vi "add setting.vi"(6 "replace if found?(T)":bool, 8 "error in (no error)":errorcluster, 9 "user settings":variant, 10 "id":string, 11 "DSFConfiguration in":refnum<class "DSFConfiguration.lvclass">) -> (0 "error out":errorcluster, 1 "found?":bool, 3 "DSFConfiguration out":refnum<class "DSFConfiguration.lvclass">)   [LabVIEW 2017, in "DSFConfiguration.lvclass"]
uses:
  DSFConfiguration.lvclass
  DSFConfiguration.lvclass/DSFConfiguration.ctl
  DSFPluginSettings/DSFPluginSettings.lvclass
  <vilib>/Utility/error.llb/Error Cluster From Error Code.vi
  <vilib>/ErrorRing/Error Ring.xnode
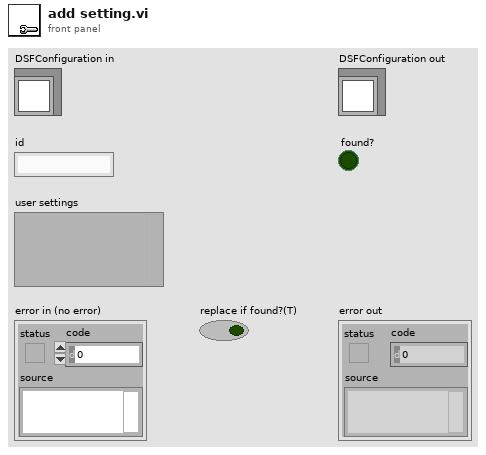
[diagram p1: front panel]
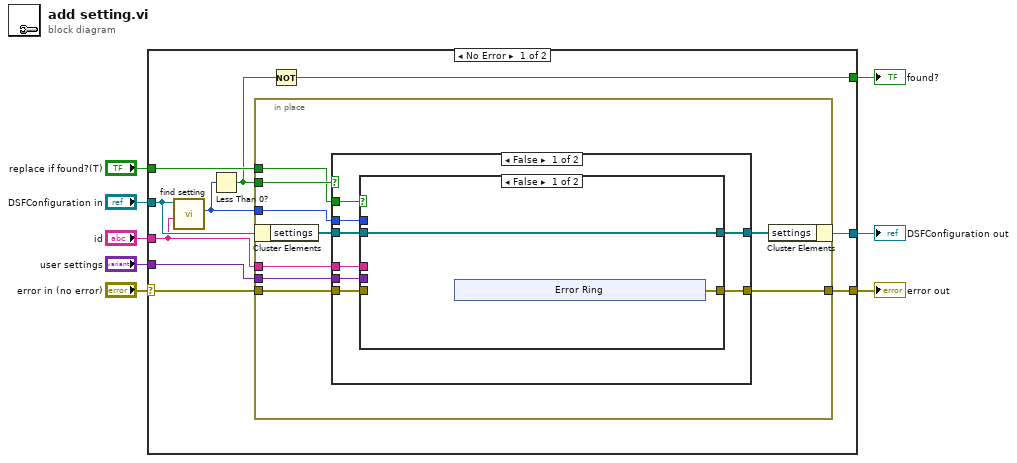
[diagram p0: block diagram]
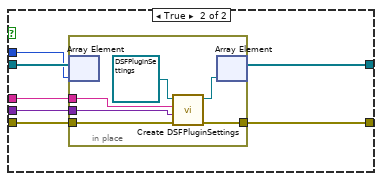
[diagram p2: hidden frame]
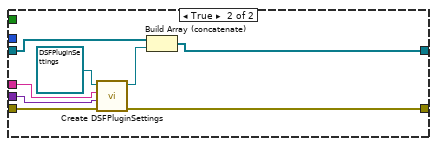
[diagram p3: hidden frame]
diagram:
  n1 = case shown="No Error" "error in (no error)" {
    selector: "error in (no error)" -> [w12 w64]
    tunnel: [w11 w64] -> w7
    tunnel: [w15 w63] -> w5
    tunnel: "DSFConfiguration in" -> [w18 w63]
    tunnel: "replace if found?(T)" -> [w17 _]
    tunnel: "id" -> [w14 _]
    tunnel: "user settings" -> [w13 _]
    tunnel: [w9 _] -> w1
    frame No Error {
      n2 = call "find setting.vi"("settings id"=w14, "DSFConfiguration in"=w18) -> ("index"=w16:i32)  [unwired: 9 in]
      n3 = Less Than 0?(x=w16) -> (x < 0?=w10:bool)
      n4 = in-place {
        in-place-border: w10 -> [w26]
        in-place-border: w14 -> [w25]
        in-place-border: w17 -> [w23]
        in-place-border: w16 -> [w22]
        in-place-border: w13 -> [w21]
        in-place-border: w12 -> [w20]
        in-place-border: [w19] -> w11
        n5 = in-place-cluster #1(w18) -> ("settings"=w27:refnum<class "DSFPluginSettings.lvclass">[])
        n6 = case shown="False" w26 {
          tunnel: w27 -> [w35 w62]
          tunnel: w25 -> [w32 w59]
          tunnel: [w31 w61] -> w24
          tunnel: w23 -> [w34 _]
          tunnel: w22 -> [w33 _]
          tunnel: w21 -> [w30 w58]
          tunnel: w20 -> [w29 w57]
          tunnel: [w28 w55] -> w19
          frame False {
            n7 = case shown="False" w34 {
              tunnel: w35 -> [w37 w48]
              tunnel: w33 -> [_ w47]
              tunnel: w32 -> [_ w46]
              tunnel: [w37 w45] -> w31
              tunnel: w30 -> [_ w44]
              tunnel: w29 -> [_ w43]
              tunnel: [w36 w42] -> w28
              frame False {
                n8 = xnode "Error Ring"() -> ("error out"=w36:errorcluster)
              }
              frame True {
                n9 = in-place {
                  in-place-border: w46 -> [w53]
                  in-place-border: w44 -> [w52]
                  in-place-border: w43 -> [w50]
                  in-place-border: [w49] -> w42
                  n10 = in-place-array #2(w48, w47) -> ()  [unwired: 1 out]
                  n11 = call "Create DSFPluginSettings.vi"("error in (no error)"=w50, "user settings"=w52, "id"=w53, "DSFPluginSettings in"=refnum<class "DSFPluginSettings.lvclass"> refnum) -> ("error out"=w49:errorcluster, "DSFPluginSettings out"=w51:refnum<class "DSFPluginSettings.lvclass">)  [unwired: 6 in]
                  n12 = in-place-array #2(w51) -> (w45:refnum<class "DSFPluginSettings.lvclass">[])  [unwired: 1 out]
                }
              }
            }
          }
          frame True {
            n13 = call "Create DSFPluginSettings.vi"("error in (no error)"=w57, "user settings"=w58, "id"=w59, "DSFPluginSettings in"=refnum<class "DSFPluginSettings.lvclass"> refnum) -> ("error out"=w55:errorcluster, "DSFPluginSettings out"=w56:refnum<class "DSFPluginSettings.lvclass">)  [unwired: 6 in]
            n14 = Build Array (concatenate)(w62, w56) -> (w61:refnum<class "DSFPluginSettings.lvclass">[])
          }
        }
        n15 = in-place-cluster #1("settings"=w24) -> (w15:refnum<class "DSFConfiguration.lvclass">)
      }
      n16 = Not(x=w10) -> (.not. x?=w9:bool)
    }
    frame Error {
    }
  }
  "error out" <- w7
  "DSFConfiguration out" <- w5
  "found?" <- w1
